vi "Translation_Integration2.vi"(0 "acc":dbl[](array[numeric]), 1 "V(i) in":dbl[](array[numeric]), 2 "latd(i)":dbl, 3 "lon(i) [rad]":dbl, 4 "alt(i) [m]":dbl, 5 "dt [s]":dbl) -> (14 "position":dbl[](array[numeric]), 15 "position ECEF (i)":dbl[](array[numeric]), 17 "L_C":dbl, 19 "Velocity":dbl[](array[numeric]))   [LabVIEW 2017]
uses:
  <vilib>/Analysis/baseanly.llb/Real A x B.vi
  <vilib>/Analysis/Matrix/Numeric/Conversions/Array To Matrix - RA2.vi
  <vilib>/Analysis/Matrix/Numeric/Conversions/Array To Matrix - RA.vi
  <vilib>/Analysis/Matrix/Numeric/Conversions/Matrix To Array - RM.vi
  <vilib>/Analysis/Matrix/NI_Matrix.lvlib
  <vilib>/Analysis/NI_AALBase.lvlib
panel:
  out "appended array":dbl[](array[numeric])
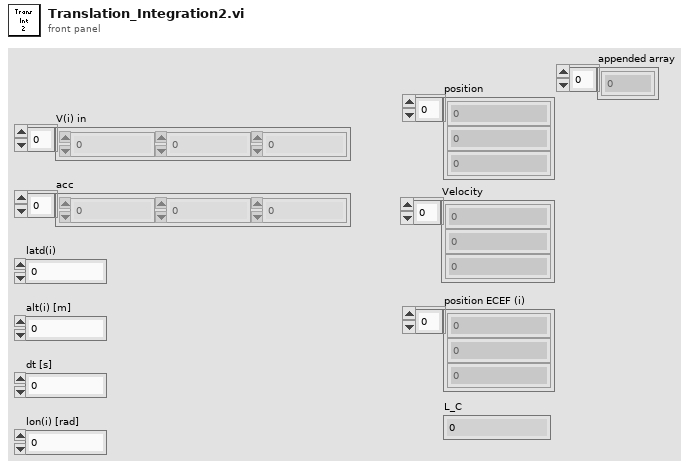
[diagram p1: front panel]
types:
  T1 = typedef "NI_Matrix.lvlib/RealMatrix.ctl" = dbl[][]
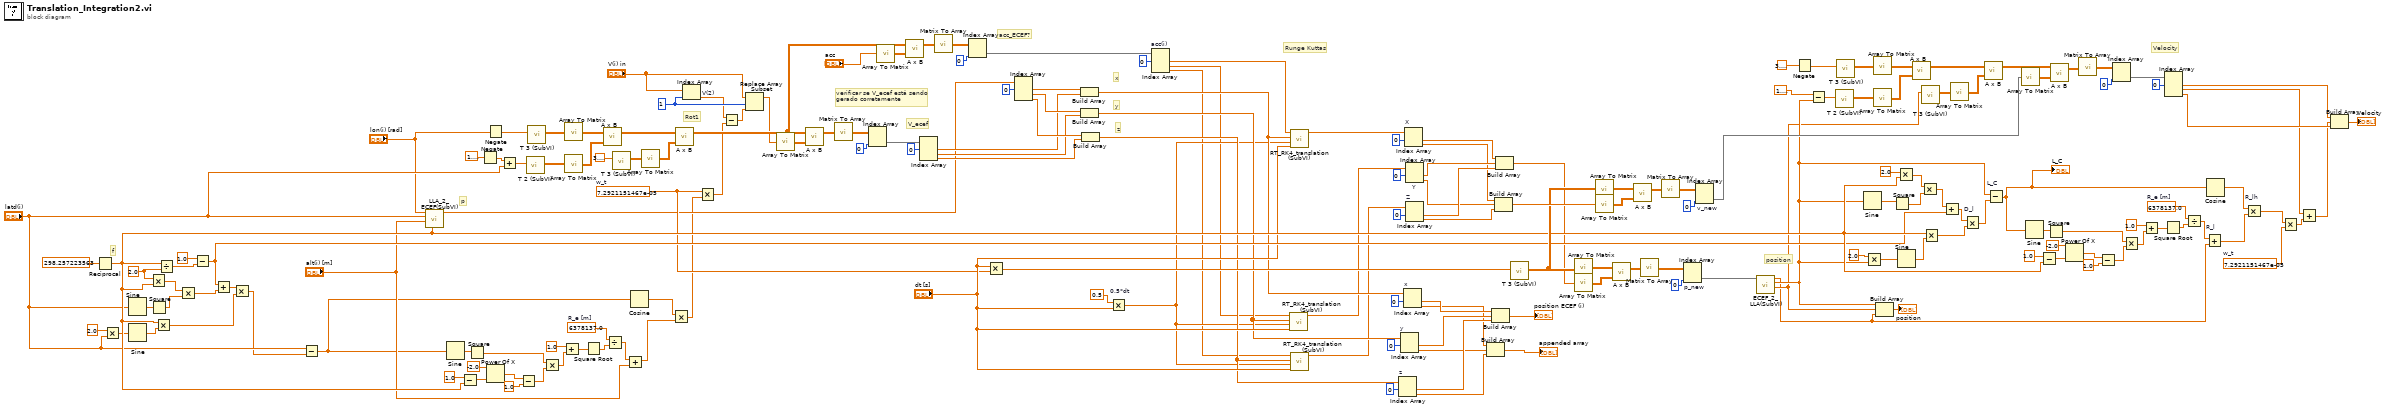
[diagram p0: block diagram]
diagram:
  w181 = 7.2921151467e-05  # w_t
  w148 = 6378137.0  # R_e [m]
  w113 = 7.2921151467e-05  # w_t
  w85 = 1 ("index")
  w40 = 2.0 ("x")
  w58 = 6378137.0  # R_e [m]
  # "Runge Kuttas"
  # "Velocity"
  # "position"
  # "z"
  # "y"
  # "x"
  # "acc_ECEF?"
  # "verificar se V_ecef está sendo \ngerado corretamente"
  # "V_ecef"
  # "Rot1"
  # "p"
  # "f"
  n1 = Reciprocal(x=298.257223563) -> (1/x=w151:dbl)
  n2 = Multiply(x=2.0, y="latd(i)") -> (x*y=w34:dbl)
  n3 = Sine(x="latd(i)") -> (sin(x)=w36:dbl)
  n4 = Sine(x=w34) -> (sin(x)=w35:dbl)
  n5 = Multiply(x=w40, y=w151) -> (x*y=w37:dbl)
  n6 = Square(x=w36) -> (x^2=w38:dbl)
  n7 = Multiply(x=w151, y=w35) -> (x*y=w44:dbl)
  n8 = Divide(x=w151, y=w40) -> (x/y=w41:dbl)
  n9 = Multiply(x=w37, y=w38) -> (x*y=w39:dbl)
  n10 = Subtract(x=1.0, y=w41) -> (x-y=w150:dbl)
  n11 = Add(x=w150, y=w39) -> (x+y=w43:dbl)
  n12 = Multiply(x=w43, y=w44) -> (x*y=w45:dbl)
  n13 = Subtract(x="latd(i)", y=w45) -> (x-y=w62:dbl)
  n14 = call "LLA_2_ECEF(SubVI).vi"("f"=w151, "alt(i) [m]"="alt(i) [m]", "latd(i)"="latd(i)", "lon(i)"="lon(i) [rad]") -> ("position"=w101:dbl[])  [unwired: 7 in]
  n15 = Sine(x=w62) -> (sin(x)=w46:dbl)
  n16 = Subtract(x=1.0, y=w151) -> (x-y=w49:dbl)
  n17 = Square(x=w46) -> (x^2=w52:dbl)
  n18 = Negate(x=1.5707963267948966) -> (-x=w70:dbl)
  n19 = Power Of X(1:w49, 2:-2.0 ("y")) -> (0:w51:dbl)
  n20 = Negate(x="lon(i) [rad]") -> (-x=w67:dbl)
  n21 = Add(x=w70, y="latd(i)") -> (x+y=w72:dbl)
  n22 = Subtract(x=w51, y=1.0 ("x")) -> (x-y=w53:dbl)
  n23 = call "T 2 (SubVI).vi"("arg"=w72) -> ("matrix"=w76:dbl[][])  [unwired: 10 in]
  n24 = call "T 3 (SubVI).vi"("arg"=w67) -> ("matrix"=w75:dbl[][])  [unwired: 10 in]
  n25 = Multiply(x=w52, y=w53) -> (x*y=w54:dbl)
  n26 = Add(x=1.0, y=w54) -> (x+y=w56:dbl)
  n27 = call-poly <vilib>:"Array To Matrix.vi"("Real 2D Array"=w75) -> ("Real Matrix"=w74:T1)
  n28 = call-poly <vilib>:"Array To Matrix.vi"("Real 2D Array"=w76) -> ("Real Matrix"=w73:T1)
  n29 = Square Root(x=w56) -> (sqrt(x)=w57:dbl)
  n30 = call-poly <vilib>:"A x B.vi"("B"=w73, "A"=w74) -> ("A x B"=w79:T1)  [unwired: 1 out]
  n31 = Divide(x=w58, y=w57) -> (x/y=w59:dbl)
  n32 = call "T 3 (SubVI).vi"("arg"=3.141592653589793) -> ("matrix"=w80:dbl[][])  [unwired: 10 in]
  n33 = Add(x=w59, y="alt(i) [m]") -> (x+y=w61:dbl)
  n34 = Cosine(x=w62) -> (cos(x)=w60:dbl)
  n35 = call-poly <vilib>:"Array To Matrix.vi"("Real 2D Array"=w80) -> ("Real Matrix"=w78:T1)
  n36 = Multiply(x=w60, y=w61) -> (x*y=w81:dbl)
  n37 = call-poly <vilib>:"A x B.vi"("B"=w78, "A"=w79) -> ("A x B"=w93:T1)  [unwired: 1 out]
  n38 = Index Array "V(2)"(array="V(i) in", index=w85) -> (element=w82:dbl)
  n39 = Multiply(x=w113, y=w81) -> (x*y=w83:dbl)
  n40 = Subtract(x=w82, y=w83) -> (x-y=w86:dbl)
  n41 = Replace Array Subset(array="V(i) in", new element=w86, index=w85) -> (w87:dbl[])
  n42 = call-poly <vilib>:"Array To Matrix.vi"("Real 1D Array"=w87) -> ("Real Matrix (Column Vector)"=w84:T1)
  n43 = call-poly <vilib>:"A x B.vi"("B"=w84, "A"=w93) -> ("A x B"=w90:T1)  [unwired: 1 out]
  n44 = call-poly <vilib>:"Matrix To Array.vi"("Real Matrix"=w90) -> ("Real 2D Array"=w88:dbl[][])
  n45 = Index Array(array=w88, index (col)=0 ("index (row)")) -> (element=w99:dbl[])  [unwired: 1 in]
  n46 = call-poly <vilib>:"Array To Matrix.vi"("Real 1D Array"="acc") -> ("Real Matrix (Column Vector)"=w92:T1)
  n47 = call-poly <vilib>:"A x B.vi"("B"=w92, "A"=w93) -> ("A x B"=w94:T1)  [unwired: 1 out]
  n48 = Index Array(array=w99, index #1=0 ("index")) -> (element #1=w102:dbl, element #2=w104:dbl, element #3=w106:dbl)  [unwired: 2 in]
  n49 = call-poly <vilib>:"Matrix To Array.vi"("Real Matrix"=w94) -> ("Real 2D Array"=w95:dbl[][])
  n50 = Index Array(array=w95, index (col)=0 ("index (row)")) -> (element=w107:dbl[])  [unwired: 1 in]
  n51 = Multiply(x="dt [s]", y=w113) -> (x*y=w118:dbl)
  n52 = Index Array(array=w101, index #1=0 ("index")) -> (element #1=w100:dbl, element #2=w103:dbl, element #3=w105:dbl)  [unwired: 2 in]
  n53 = Build Array(w100, w102) -> (w109:dbl[])
  n54 = Build Array(w103, w104) -> (w110:dbl[])
  n55 = Build Array(w105, w106) -> (w111:dbl[])
  n56 = Multiply "0.5*dt"(x=0.5, y="dt [s]") -> (x*y=w17:dbl)
  n57 = Index Array "acc(i)"(array=w107, index #1=0 ("index")) -> (element #1=w14:dbl, element #2=w15:dbl, element #3=w16:dbl)  [unwired: 2 in]
  n58 = call "RT_RK4_translation (SubVI).vi"("dt"="dt [s]", "dt*0.5"=w17, "x(i)"=w110, "acc"=w15) -> ("x(i+1)"=w27:dbl[])  [unwired: 7 in]
  n59 = call "RT_RK4_translation (SubVI).vi"("dt"="dt [s]", "dt*0.5"=w17, "x(i)"=w109, "acc"=w14) -> ("x(i+1)"=w28:dbl[])  [unwired: 7 in]
  n60 = call "RT_RK4_translation (SubVI).vi"("dt"="dt [s]", "dt*0.5"=w17, "x(i)"=w111, "acc"=w16) -> ("x(i+1)"=w26:dbl[])  [unwired: 7 in]
  n61 = Index Array "z"(array=w111, index #1=0 ("index")) -> (element #1=w66:dbl, element #2=w63:dbl)  [unwired: 1 in]
  n62 = Index Array "y"(array=w110, index #1=0 ("index")) -> (element #1=w65:dbl, element #2=w22:dbl)  [unwired: 1 in]
  n63 = Index Array "x"(array=w109, index #1=0 ("index")) -> (element #1=w64:dbl, element #2=w21:dbl)  [unwired: 1 in]
  n64 = Index Array "X"(array=w28, index #1=0 ("index")) -> (element #1=w115:dbl, element #2=w29:dbl)  [unwired: 1 in]
  n65 = Index Array "Y"(array=w27, index #1=0 ("index")) -> (element #1=w116:dbl, element #2=w30:dbl)  [unwired: 1 in]
  n66 = Index Array "Z"(array=w26, index #1=0 ("index")) -> (element #1=w117:dbl, element #2=w31:dbl)  [unwired: 1 in]
  n67 = Build Array(w21, w22, w63) -> (→"appended array":dbl[])
  n68 = Build Array(w64, w65, w66) -> (→"position ECEF (i)":dbl[])
  n69 = Build Array(w29, w30, w31) -> (w161:dbl[])
  n70 = Build Array(w115, w116, w117) -> (w123:dbl[])
  n71 = call "T 3 (SubVI).vi"("arg"=w118) -> ("matrix"=w160:dbl[][])  [unwired: 10 in]
  n72 = call-poly <vilib>:"Array To Matrix.vi"("Real 2D Array"=w160) -> ("Real Matrix"=w119:T1)
  n73 = call-poly <vilib>:"Array To Matrix.vi"("Real 1D Array"=w123) -> ("Real Matrix (Column Vector)"=w120:T1)
  n74 = call-poly <vilib>:"Array To Matrix.vi"("Real 2D Array"=w160) -> ("Real Matrix"=w159:T1)
  n75 = call-poly <vilib>:"Array To Matrix.vi"("Real 1D Array"=w161) -> ("Real Matrix (Column Vector)"=w158:T1)
  n76 = call-poly <vilib>:"A x B.vi"("B"=w120, "A"=w119) -> ("A x B"=w121:T1)  [unwired: 1 out]
  n77 = call-poly <vilib>:"A x B.vi"("B"=w158, "A"=w159) -> ("A x B"=w156:T1)  [unwired: 1 out]
  n78 = call-poly <vilib>:"Matrix To Array.vi"("Real Matrix"=w121) -> ("Real 2D Array"=w6:dbl[][])
  n79 = call-poly <vilib>:"Matrix To Array.vi"("Real Matrix"=w156) -> ("Real 2D Array"=w157:dbl[][])
  n80 = Index Array "p_new"(array=w6, index (col)=0 ("index (row)")) -> (element=w124:dbl[])  [unwired: 1 in]
  n81 = Index Array "v_new"(array=w157, index (col)=0 ("index (row)")) -> (element=w178:dbl[])  [unwired: 1 in]
  n82 = call "ECEF_2_LLA(SubVI).vi"("p_new"=w124) -> ("lon"=w10:dbl, "latd"=w11:dbl, "altd"=w9:dbl)  [unwired: 8 in]
  n83 = Negate(x=3.141592653589793) -> (-x=w162:dbl)
  n84 = Subtract(x=1.5707963267948966, y=w11) -> (x-y=w163:dbl)
  n85 = call "T 2 (SubVI).vi"("arg"=w163) -> ("matrix"=w167:dbl[][])  [unwired: 10 in]
  n86 = call "T 3 (SubVI).vi"("arg"=w162) -> ("matrix"=w166:dbl[][])  [unwired: 10 in]
  n87 = Sine(x=w11) -> (sin(x)=w128:dbl)
  n88 = Multiply(x=2.0, y=w11) -> (x*y=w126:dbl)
  n89 = call-poly <vilib>:"Array To Matrix.vi"("Real 2D Array"=w166) -> ("Real Matrix"=w165:T1)
  n90 = call-poly <vilib>:"Array To Matrix.vi"("Real 2D Array"=w167) -> ("Real Matrix"=w164:T1)
  n91 = Build Array(w11, w10, w9) -> (→"position":dbl[])
  n92 = Square(x=w128) -> (x^2=w131:dbl)
  n93 = Multiply(x=2.0, y=w151) -> (x*y=w130:dbl)
  n94 = Sine(x=w126) -> (sin(x)=w127:dbl)
  n95 = call-poly <vilib>:"A x B.vi"("B"=w164, "A"=w165) -> ("A x B"=w169:T1)  [unwired: 1 out]
  n96 = Multiply(x=w130, y=w131) -> (x*y=w132:dbl)
  n97 = call "T 3 (SubVI).vi"("arg"=w10) -> ("matrix"=w170:dbl[][])  [unwired: 10 in]
  n98 = Multiply(x=w151, y=w127) -> (x*y=w134:dbl)
  n99 = Add(x=w132, y=w150) -> (x+y=w133:dbl)
  n100 = call-poly <vilib>:"Array To Matrix.vi"("Real 2D Array"=w170) -> ("Real Matrix"=w168:T1)
  n101 = Multiply "D_l"(x=w133, y=w134) -> (x*y=w135:dbl)
  n102 = call-poly <vilib>:"A x B.vi"("B"=w168, "A"=w169) -> ("A x B"=w177:T1)  [unwired: 1 out]
  n103 = Subtract "L_C"(x=w11, y=w135) -> (x-y=w152:dbl)
  "L_C" <- w152
  n104 = call-poly <vilib>:"Array To Matrix.vi"("Real 1D Array"=w178) -> ("Real Matrix (Column Vector)"=w172:T1)
  n105 = Sine(x=w152) -> (sin(x)=w136:dbl)
  n106 = Subtract(x=1.0, y=w151) -> (x-y=w139:dbl)
  n107 = Square(x=w136) -> (x^2=w142:dbl)
  n108 = call-poly <vilib>:"A x B.vi"("B"=w172, "A"=w177) -> ("A x B"=w174:T1)  [unwired: 1 out]
  n109 = Power Of X(1:w139, 2:-2.0 ("y")) -> (0:w141:dbl)
  n110 = call-poly <vilib>:"Matrix To Array.vi"("Real Matrix"=w174) -> ("Real 2D Array"=w179:dbl[][])
  n111 = Subtract(x=w141, y=1.0 ("x")) -> (x-y=w143:dbl)
  n112 = Index Array(array=w179, index (col)=0 ("index (row)")) -> (element=w176:dbl[])  [unwired: 1 in]
  n113 = Multiply(x=w142, y=w143) -> (x*y=w144:dbl)
  n114 = Add(x=1.0, y=w144) -> (x+y=w146:dbl)
  n115 = Square Root(x=w146) -> (sqrt(x)=w147:dbl)
  n116 = Index Array(array=w176, index #1=0 ("index")) -> (element #1=w183:dbl, element #2=w4:dbl, element #3=w5:dbl)  [unwired: 2 in]
  n117 = Divide(x=w148, y=w147) -> (x/y=w149:dbl)
  n118 = Add "R_l"(x=w149, y=w9) -> (x+y=w154:dbl)
  n119 = Cosine(x=w152) -> (cos(x)=w153:dbl)
  n120 = Multiply "R_lh"(x=w153, y=w154) -> (x*y=w180:dbl)
  n121 = Multiply(x=w180, y=w181) -> (x*y=w182:dbl)
  n122 = Add(x=w4, y=w182) -> (x+y=w3:dbl)
  n123 = Build Array(w183, w3, w5) -> (→"Velocity":dbl[])
